vi "Add Items.vi"(8 "error in (no error)":errorcluster, 9 "Reset":bool, 10 "Items":string[](array[string]), 11 "Sequence Element in":refnum<class "Sequence Element.lvclass">) -> (0 "error out":errorcluster, 3 "Sequence Element out":refnum<class "Sequence Element.lvclass">)   [LabVIEW 2016, in "Sequence Element.lvclass"]
uses:
  Sequence Element.lvclass
  Sequence Element.lvclass/Sequence Element.ctl
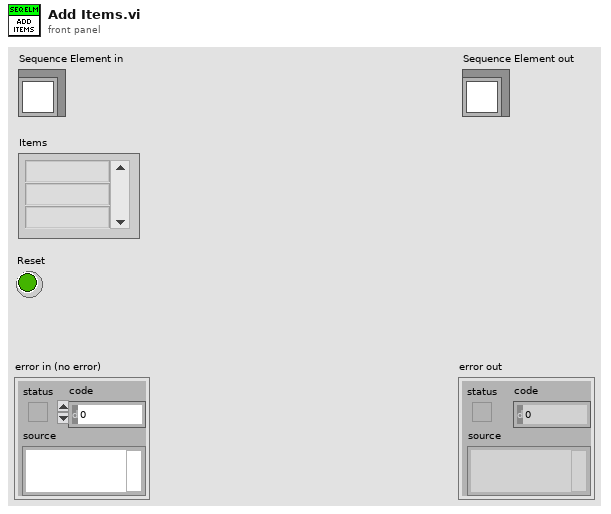
[diagram p1: front panel]
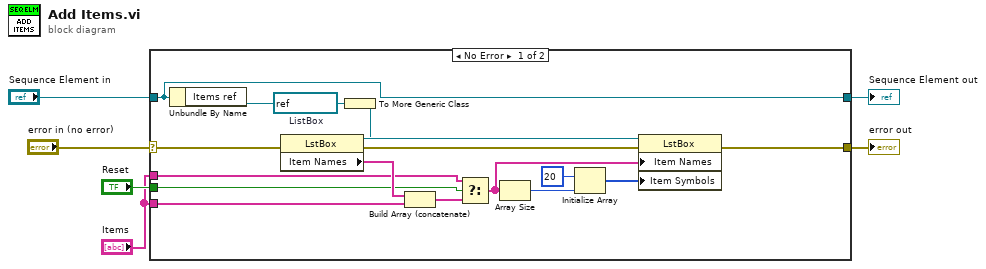
[diagram p0: block diagram]
diagram:
  n1 = case shown="No Error" "error in (no error)" {
    selector: "error in (no error)" -> [w11 w25]
    tunnel: [w10 w25] -> w5
    tunnel: [w23 w24] -> w3
    tunnel: "Sequence Element in" -> [w23 w24]
    tunnel: "Reset" -> [w20 _]
    tunnel: "Items" -> [w21 _]
    tunnel: "Items" -> [w19 _]
    frame No Error {
      w7 = refnum<vi> refnum  # ListBox
      n2 = Unbundle By Name(w23) -> ("Items ref"=w8:refnum<vi>)
      n3 = To More Generic Class(target class=w7, reference=w8) -> (generic class reference=w9:refnum<vi>)
      n4 = property class="LstBox"(reference=w9, error in=w11) -> (reference out=w17:refnum<vi>, error out=w12:errorcluster, "Item Names"=w22:string[])
      n5 = Build Array (concatenate)(w22, w21) -> (w18:string[])
      n6 = Select(t=w19, s=w20, f=w18) -> (s? t:f=w16:string[])
      n7 = Array Size(array=w16) -> (size(s)=w15:i32)
      n8 = Initialize Array(20, w15) -> (w13:i32[])
      n9 = property class="LstBox"(reference=w17, error in=w12, "Item Names"=w16, "Item Symbols"=w13) -> (error out=w10:errorcluster)  [unwired: 1 out]
    }
    frame Error {
    }
  }
  "error out" <- w5
  "Sequence Element out" <- w3
